vi "TDTSyn-Rewrite CAR Matrices.vi"(0 "URL":string="http://localhost:24414", 5 "ChanCount":i32[](array[numeric]), 7 "Refs":refnum<vi>[](array[refnum]), 11 "error in (no error)":errorcluster) -> (15 "error out":errorcluster)   [LabVIEW 2020]
uses:
  CAR Control/CAR Control.xctl
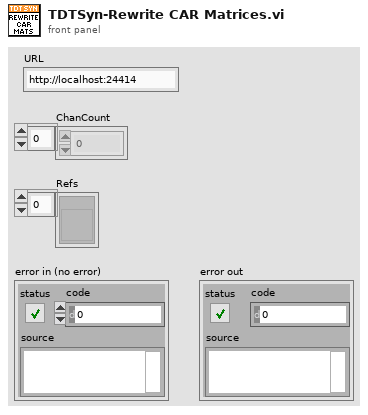
[diagram p1: front panel]
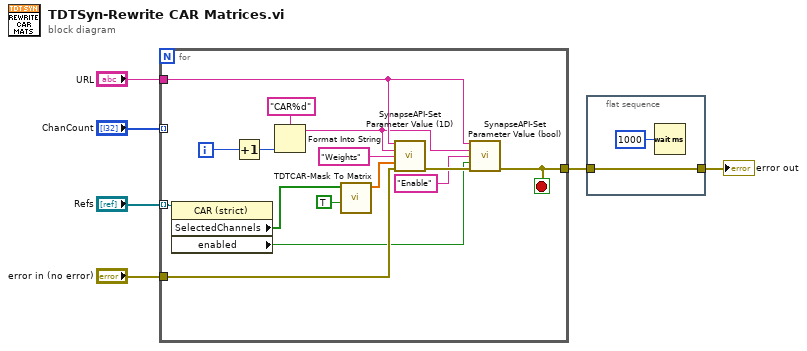
[diagram p0: block diagram]
diagram:
  n1 = for {
    tunnel: "ChanCount" -> [_] mode=indexing
    tunnel: "Refs" -> [w18] mode=indexing
    tunnel: "error in (no error)" -> [w14]
    tunnel: [w11] -> w2
    tunnel: "URL" -> [w10]
    i -> [w16]
    stop <- w11 stop-if-true
    n2 = property class="CAR (strict)"(reference=w18) -> ("SelectedChannels"=w13:bool[], "enabled"=w7:bool)  [unwired: 1 in, 2 out]
    n3 = Increment(x=w16) -> (x+1=w15:i32)
    n4 = Format Into String(format string="CAR%d" ("Gizmo"), w15) -> (resulting string=w9:string)  [unwired: 2 in, 1 out]
    n5 = call "TDTCAR-Mask To Matrix.vi"("Enable?"=TRUE, "Mask In"=w13) -> ("CAR Matrix"=w20:dbl[])  [unwired: 8 in, 1 out]
    n6 = call "SynapseAPI-Set Parameter Value (1D).vi"("URL"=w10, "Gizmo"=w9, "Parameter"="Weights" ("Target"), "Values"=w20, "error in (no error)"=w14) -> ("error out"=w12:errorcluster)  [unwired: 10 in]
    n7 = call "SynapseAPI-Set Parameter Value (bool).vi"("URL"=w10, "Gizmo"=w9, "Parameter"="Enable", "Value"=w7, "error in (no error)"=w12) -> ("error out"=w11:errorcluster)  [unwired: 10 in]
  }
  n8 = flat-sequence {
    tunnel: w2 -> [w23]
    tunnel: [w23] -> w1
    frame #0 {
      n9 = Wait (ms)(milliseconds to wait=u32 1000) -> ()  [unwired: 1 out]
    }
  }
  "error out" <- w1
